vi "maszyna_stanu.vi"() -> ()   [LabVIEW 2018]
uses:
  <vilib>/sound2/lvsound2.llb/Sound Data Format.ctl
  stany.ctl
  <vilib>/sound2/lvsound2.llb/Sampling Mode.ctl
  <vilib>/sound2/lvsound2.llb/Sound Input Read (DBL).vi
panel:
  in  "stop":bool
  out "Numeric":i32
  in  "sound format":T1={"sample rate (S/s)"=22050.0, "number of channels"=2, "bits per sample"=16}
  in  "number of samples/ch":i32=100000
  out "Waveform Graph":waveform(dbl)[](graph)
  in  "PLAY":bool
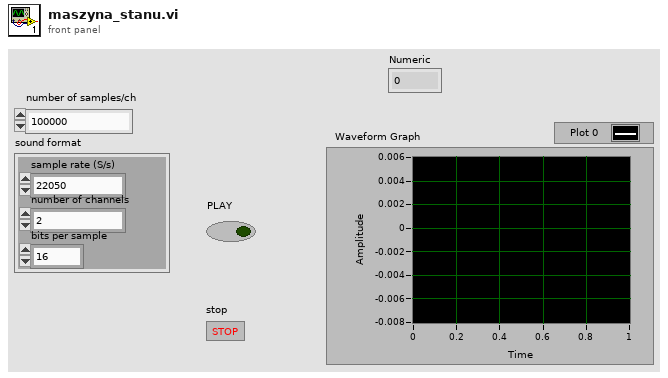
[diagram p1: front panel]
types:
  T1 = typedef "Sound Data Format.ctl" = cluster{"sample rate (S/s)":dbl, "number of channels":i32, "bits per sample":i32}
  T2 = typedef "stany.ctl" = enum16{"Idle", "Initialization", "Acquisition", "End"}
  T3 = typedef "Sampling Mode.ctl" = i32
  T4 = typedef "Sound Input Task ID.ctl" = u32
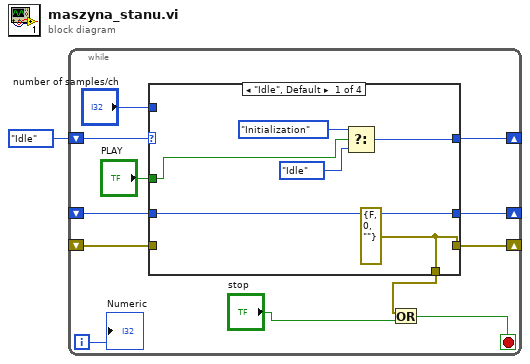
[diagram p0: block diagram]
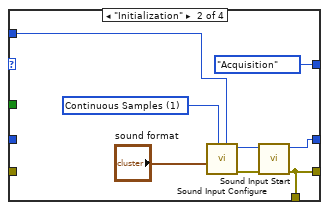
[diagram p2: hidden frame]
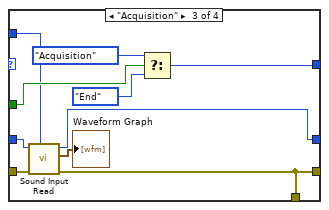
[diagram p3: hidden frame]
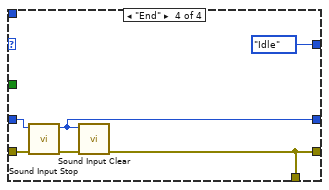
[diagram p4: hidden frame]
diagram:
  n1 = while {
    shift-right: [w12] -> _
    shift-left: stany."Idle" -> [w13]
    shift-right: [w9] -> _
    shift-left: _ -> [w8]
    shift-right: [w10] -> _
    shift-left: _ -> [w7]
    i -> [w6]
    stop <- w2 stop-if-true
    n2 = case shown="\"Idle\", Default" w13 {
      tunnel: [w17 stany."Acquisition" w34 stany."Idle"] -> w12
      tunnel: "PLAY" -> [w16 _ w37 _]
      tunnel: [w15 w24 w31 w39] -> w10
      tunnel: [w14 w20 w28 w38] -> w9
      tunnel: w8 -> [_ _ w32 w41]
      tunnel: w7 -> [w15 _ w33 w40]
      tunnel: "number of samples/ch" -> [_ w21 w29 _]
      tunnel: [w14 w20 w28 w38] -> w4
      frame "Idle", Default {
        w14 = errorcluster {"status"=FALSE, "code"=0, "source"=""} ("error out")
        n3 = Select(t=stany."Initialization", s=w16, f=stany."Idle") -> (s? t:f=w17:T2)
      }
      frame "Initialization" {
        w22 = T3 1 items=["Finite Samples", "Continuous Samples"] ("sample mode")
        n4 = call <vilib>:"Sound Input Configure.vi"("number of samples/ch"=w21, "sample mode"=w22, "sound format"="sound format") -> ("error out"=w26:errorcluster, "task ID"=w27:T4)  [unwired: 7 in]
        n5 = call <vilib>:"Sound Input Start.vi"("error in (no error)"=w26, "task ID"=w27) -> ("error out"=w20:errorcluster, "task ID out"=w24:T4)  [unwired: 8 in]
      }
      frame "Acquisition" {
        n6 = call-poly <vilib>:"Sound Input Read.vi"("number of samples/ch"=w29, "error in (no error)"=w32, "task ID"=w33) -> ("error out"=w28:errorcluster, "data"=→"Waveform Graph":waveform(dbl)[], "task ID out"=w31:T4)  [unwired: 6 in]
        n7 = Select(t=stany."Acquisition", s=w37, f=stany."End") -> (s? t:f=w34:T2)
      }
      frame "End" {
        n8 = call <vilib>:"Sound Input Stop.vi"("error in (no error)"=w41, "task ID"=w40) -> ("error out"=w43:errorcluster, "task ID out"=w39:T4)  [unwired: 8 in]
        n9 = call <vilib>:"Sound Input Clear.vi"("error in (no error)"=w43, "task ID"=w39) -> ("error out"=w38:errorcluster)  [unwired: 9 in]
      }
    }
    n10 = Or(x=w4, y="stop") -> (x .or. y?=w2:bool)
    "Numeric" <- w6
  }
